vi "subpanel.vi"(5 "Panel Transparent":bool, 7 "Wait Until Done":bool, 8 "error in":errorcluster, 10 "Vi":path=path "C:/CT/Software/Panel/Configuration/GeneralConfigurationView.vi", 11 "SubPanel":refnum<vi>) -> (0 "error out":errorcluster, 2 "NextScreen":T1=enum."Config", 3 "ControlValues":cluster{"Name":string, "Variant Data":variant}[](array[cluster]))   [LabVIEW 2019]
uses:
  Telas.ctl
  Users/Nicole/Downloads/a/ims-desktop/Variaveis/CodOrder.vi
  Users/Nicole/Downloads/a/ims-desktop/Variaveis/SubPanelReference.vi
panel:
  out "Stop":bool=TRUE
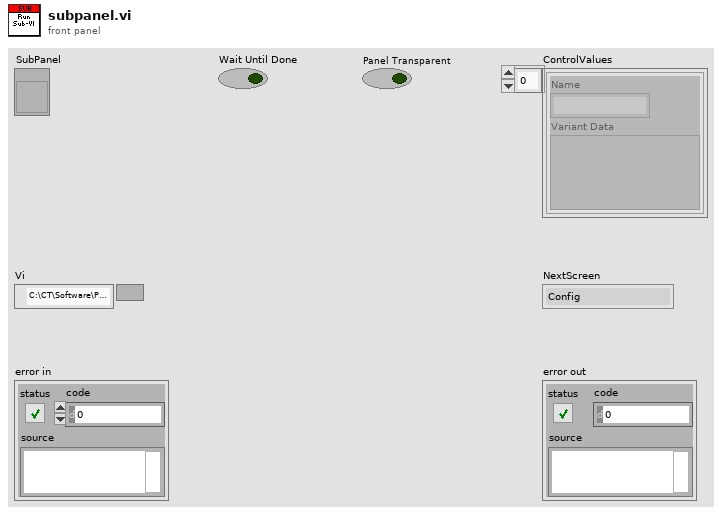
[diagram p1: front panel]
types:
  T1 = typedef "Telas.ctl" = enum16{"Selecao", "Config", "Medicao"}
  T2 = typedef "Telas.ctl" = enum16{"Operator", "MeasureFrameTestCommunication", "MeasureFrame", "CNCLoadProgram", "RotorBrokenBars", "Configuration", "MeasureFramePreparation", "WindingLabel", "OtherLabel", "InsulationTapeLabel", "WindingSpecialLabel", "GCF", "AssemblyWindingLabel", "Press", "ThermalProtectorLabel", "Traceability", "MeasureFrameProductionOrder", "MeasureFrameStandardEquipment", "MeasureFrameReferentiate", "LabelScanner", "Alerts", "ProductImages", "QGA", "RotorExternalDiameter", "ComponentRegistration", "WindingInspectionInsulationTapeId", "WindingInspectionPreparation", "WindingInspectionMonitoring", "BearingStiffnessMotorIdentification", "BearingStiffnessLvdtSetup", "BearingStiffness", "WindingInspectionMeasureResistance", "BearingStiffnessManualMode", "Calibration", "PressTooling", "GageDrawing", "BalancingReportProductionOrder", "BalancingReport", "PressMeasureAndControl", "WireFaultDetectionMAG", "StatorImpregnationWeight", "MeasureCapacitance", "SpecialCover", "RegistrationOfInspectionDocuments", "BearingHouseDiameter", "HeaterTemperatureRecord", "PackageLength", "Cnc", "BadgeRegistration", "SpecialFrame", "TerminalBoxFitting", "CoordinateMeasuringMachineDataConversion", "Checklist", "FrameCoverFit", "ShaftGrindingInspection", "ShaftBearingPress", "RotorHeatTreatment", "PressingMeasureBeatPulley", "MotorVisualInspection", "VacuumImpregnation", "Standards", "PaintPreparation", "Runout"}
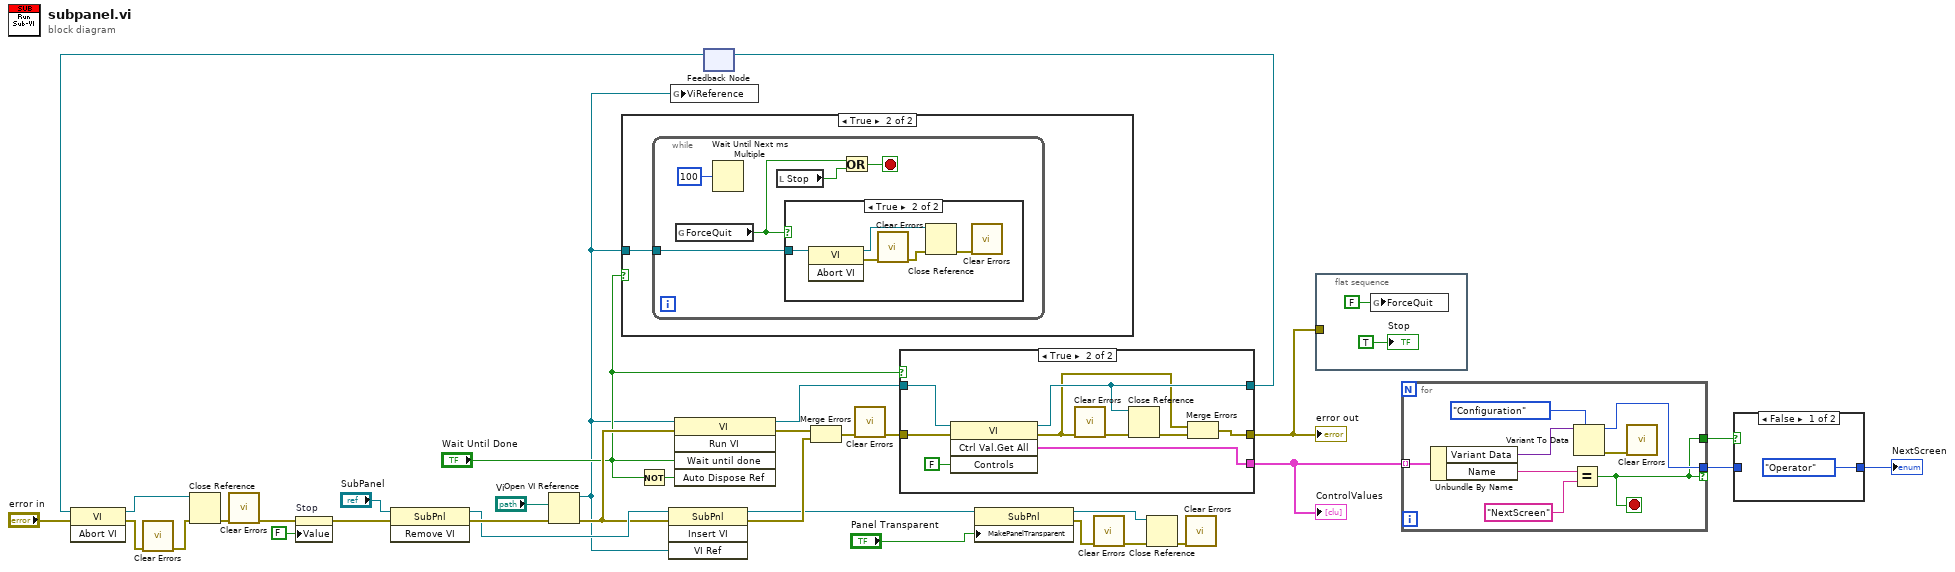
[diagram p0: block diagram]
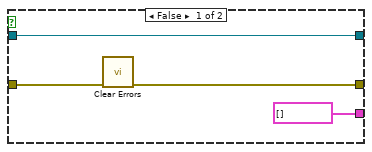
[diagram p4: hidden frame]
diagram:
  n1 = Not(x="Wait Until Done") -> (.not. x?=w19:bool)
  n2 = feedback #1() -> (w30:refnum<vi>)  [unwired: 1 in]
  n3 = invoke class="VI" method="Abort VI"(reference=w30, error in="error in") -> (reference out=w29:refnum<vi>, error out=w6:errorcluster)  [unwired: 1 in, 1 out]
  n4 = call <vilib>:"Clear Errors.vi"("error in (no error)"=w6) -> ("error out"=w5:errorcluster)  [unwired: 5 in, 1 out]
  n5 = Close Reference(reference=w29, error in (no error)=w5) -> (error out=w31:errorcluster)
  n6 = call <vilib>:"Clear Errors.vi"("error in (no error)"=w31) -> ("error out"=w10:errorcluster)  [unwired: 5 in, 1 out]
  n7 = property on="Stop" class="Bool (strict)"(error in=w10, "Value"=FALSE ("Stop")) -> (error out=w9:errorcluster)  [unwired: 1 in, 1 out]
  n8 = invoke on="Invoke Node" class="SubPnl" method="Remove VI"(reference="SubPanel", error in=w9) -> (reference out=w32:refnum<vi>, error out=w33:errorcluster)  [unwired: 1 in, 1 out]
  n9 = Open VI Reference(vi path="Vi", error in (no error)=w33) -> (vi reference=w7:refnum<vi>, error out=w14:errorcluster)  [unwired: 4 in]
  n10 = case shown="True" "Wait Until Done" {
    tunnel: w7 -> [_ w35]
    frame False {
    }
    frame True {
      n11 = while {
        tunnel: w35 -> [w40]
        stop <- w38 stop-if-true
        n12 = global read "CodOrder.vi" "ForceQuit"() -> (w37:bool)
        n13 = Wait Until Next ms Multiple(millisecond multiple=u32 100) -> ()  [unwired: 1 out]
        n14 = local read "Stop"() -> (w39:bool)
        n15 = case shown="True" w37 {
          tunnel: w40 -> [_ w45]
          frame False {
          }
          frame True {
            n16 = invoke class="VI" method="Abort VI"(reference=w45) -> (reference out=w43:refnum<vi>, error out=w44:errorcluster)  [unwired: 2 in, 1 out]
            n17 = call <vilib>:"Clear Errors.vi"("error in (no error)"=w44) -> ("error out"=w42:errorcluster)  [unwired: 5 in, 1 out]
            n18 = Close Reference(reference=w43, error in (no error)=w42) -> (error out=w41:errorcluster)
            n19 = call <vilib>:"Clear Errors.vi"("error in (no error)"=w41) -> ()  [unwired: 5 in, 2 out]
          }
        }
        n20 = Or(x=w37, y=w39) -> (x .or. y?=w38:bool)
      }
    }
  }
  n21 = invoke on="Invoke Node" class="SubPnl" method="Insert VI"(reference=w32, error in=w14, "VI Ref"=w7) -> (reference out=w21:refnum<vi>, error out=w27:errorcluster)  [unwired: 1 in, 2 out]
  n22 = global write "SubPanelReference.vi" "ViReference"(w7) -> ()
  n23 = invoke class="VI" method="Run VI"(reference=w7, error in=w14, "Wait until done"="Wait Until Done", "Auto Dispose Ref"=w19) -> (reference out=w24:refnum<vi>, error out=w26:errorcluster)  [unwired: 1 in, 3 out]
  n24 = Merge Errors(w26, w27) -> (w25:errorcluster)
  n25 = call <vilib>:"Clear Errors.vi"("error in (no error)"=w25) -> ("error out"=w8:errorcluster)  [unwired: 5 in, 1 out]
  n26 = case shown="True" "Wait Until Done" {
    tunnel: w8 -> [w49 w55]
    tunnel: [w48 w52] -> w12
    tunnel: w24 -> [w47 w57]
    tunnel: [w47 w53] -> w23
    tunnel: [cluster{"Name":string, "Variant Data":variant}[] [] ("Get All Control Values Variant") w56] -> w18
    frame False {
      n27 = call <vilib>:"Clear Errors.vi"("error in (no error)"=w49) -> ("error out"=w48:errorcluster)  [unwired: 5 in, 1 out]
    }
    frame True {
      n28 = invoke class="VI" method="Ctrl Val.Get All"(reference=w57, error in=w55, "Controls"=FALSE) -> (reference out=w53:refnum<vi>, error out=w50:errorcluster, "Get All Control Values Variant"=w56:cluster{"Name":string, "Variant Data":variant}[])  [unwired: 1 in, 1 out]
      n29 = call <vilib>:"Clear Errors.vi"("error in (no error)"=w50) -> ("error out"=w51:errorcluster)  [unwired: 5 in, 1 out]
      n30 = Close Reference(reference=w53, error in (no error)=w51) -> (error out=w54:errorcluster)
      n31 = Merge Errors(w50, w54) -> (w52:errorcluster)
    }
  }
  "error out" <- w12
  "ControlValues" <- w18
  n32 = feedback-in #1(w23) -> ()
  n33 = property class="SubPnl"(reference=w21, "MakePanelTransparent"="Panel Transparent") -> (reference out=w1:refnum<vi>, error out=w2:errorcluster)  [unwired: 1 in]
  n34 = call <vilib>:"Clear Errors.vi"("error in (no error)"=w2) -> ("error out"=w4:errorcluster)  [unwired: 5 in, 1 out]
  n35 = Close Reference(reference=w1, error in (no error)=w4) -> (error out=w3:errorcluster)
  n36 = call <vilib>:"Clear Errors.vi"("error in (no error)"=w3) -> ()  [unwired: 5 in, 2 out]
  n37 = flat-sequence {
    tunnel: w12 -> [_]
    frame #0 {
      n38 = global write "CodOrder.vi" "ForceQuit"(FALSE ("ForceQuit")) -> ()
      "Stop" <- TRUE
    }
  }
  n39 = for {
    tunnel: w18 -> [w68] mode=indexing
    tunnel: [w64] -> w16 if=w63
    tunnel: [w63] -> w17
    stop <- w63 stop-if-true
    n40 = Unbundle By Name(w68) -> ("Variant Data"=w61:variant, "Name"=w62:string)
    n41 = Equal?(x=w62, y="NextScreen") -> (x = y?=w63:bool)
    n42 = Variant To Data(type=Telas."Configuration" ("element"), Variant=w61) -> (data=w64:T2, error out=w66:errorcluster)  [unwired: 1 in]
    n43 = call <vilib>:"Clear Errors.vi"("error in (no error)"=w66) -> ()  [unwired: 5 in, 2 out]
  }
  n44 = case shown="False" w17 {
    tunnel: w16 -> [_ w70]
    tunnel: [Telas."Operator" ("element") w70] -> w15
    frame False {
    }
    frame True {
    }
  }
  "NextScreen" <- w15
